vi "module api test.vi"() -> ()   [LabVIEW 2013, in "scan engine tests.lvlib"]
uses:
  scan engine tests.lvlib
  configuration/Scan Engine configuration.lvclass
  execution/Scan Engine runtime.lvclass
  <vilib>/NI/Tag Bus Module Framework/channel/channel classification.ctl
  <vilib>/NI/Tag Bus/tag/Data Type.ctl
  <vilib>/Platform/TimedLoop/XDataNode/timing_clust.ctl
  <vilib>/Platform/TimedLoop/XDataNode/nitl_modes.ctl
  <vilib>/Platform/TimedLoop/XDataNode/wakeup.ctl
  <vilib>/NI/Module Timing Source/timing source/TBM timing source.lvclass
  <vilib>/platform/TimedLoop/XDataNode/XDataNode.xnode
  <vilib>/NI/Tag Bus/tag/tag descriptor.lvclass
  <vilib>/NI/Tag Bus Module Framework/channel/TBM channel.lvclass
  <vilib>/Platform/TimedLoop/XDataNode/XDNodeRunTimeDep.lvlib
panel:
  out "Numeric":i32
  in  "stop":bool
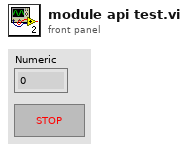
[diagram p1: front panel]
types:
  T1 = typedef "TBM channel.lvclass/channel classification.ctl" = enum16{"input data", "output data", "processing parameter", "processing result"}
  T2 = typedef "tag bus.lvlib/tag descriptor.lvclass/Data Type.ctl" = enum16{"Double", "Single", "I64", "I32", "I16", "I8", "U64", "U32", "U16", "U8", "Boolean", "String", "Array of Double", "Array of Single", "Array of I64", "Array of I32", "Array of I16", "Array of I8", "Array of U64", "Array of U32", "Array of U16", "Array of U8", "Array of Boolean", "Array of String"}
  T3 = typedef "TBM channel.lvclass/data tables.ctl" = cluster{"input data":T4, "processing parameter":T4, "processing result":T4, "output data":T4}
  T4 = typedef "tag bus.lvlib/dictionary table pair.ctl" = cluster{"data dictionary":refnum<class "data dictionary.lvclass">, "data table":T5}
  T5 = typedef "tag bus.lvlib/data table.lvlib/data table.ctl" = cluster{"Double":dbl[], "Single":sgl[], "I64":i64[], "I32":i32[], "I16":i16[], "I8":i8[], "U64":u64[], "U32":u32[], "U16":u16[], "U8":u8[], "Boolean":bool[], "String":string[], "Array of Double":cluster{"DBL Array":dbl[]}[], "Array of Single":cluster{"SGL Array":sgl[]}[], "Array of I64":cluster{"I64 Array":i64[]}[], "Array of I32":cluster{"I32 Array":i32[]}[], "Array of I16":cluster{"I16 Array":i16[]}[], "Array of I8":cluster{"I8 Array":i8[]}[], "Array of U64":cluster{"U64 Array":u64[]}[], "Array of U32":cluster{"U32 Array":u32[]}[], "Array of U16":cluster{"U16 Array":u16[]}[], "Array of U8":cluster{"U8 Array":u8[]}[], "Array of Boolean":cluster{"Boolean Array":bool[]}[], "Array of String":cluster{"String Array":string[]}[]}
  T6 = typedef "XDNodeRunTimeDep.lvlib/timing_clust.ctl" = cluster{"Expected End [f-1]":u64, "Actual End [f-1]":u64, "Finished Late? [f-1]":bool, "Expected End [i-1]":u64, "Actual End [i-1]":u64, "Finished Late? [i-1]":bool, "Expected Start [i]":u64, "Actual Start [i]":u64, "Expected Start [f]":u64, "Actual Start [f]":u64, "Source Name":string, "Structure Name":string, "Period":i64, "Deadline":i64, "Offset":i64, "Start":i64, "Priority":i32, "Timeout":i32, "Mode":T7, "Wakeup Reason":T8, "Error":errorcluster, "Source Type":string, "Secondary Source Type":string, "Global End Time":u64, "Global Start Time":u64, "Frame Duration":u64, "Iteration Duration":u64, "Assigned CPU":i32, "I/O Scan Engine Mode":u32}
  T7 = typedef "XDNodeRunTimeDep.lvlib/nitl_modes.ctl" = enum32{"No Change", "Process missed periods, maintain original phase", "Discard missed periods, maintain original phase", "Process missed periods, ignore original phase", "Discard missed periods, ignore original phase"}
  T8 = typedef "XDNodeRunTimeDep.lvlib/wakeup.ctl" = enum32{"Normal", "Aborted", "Asynchronous wakeup", "Timing source error", "Timed loop error", "Timeout"}
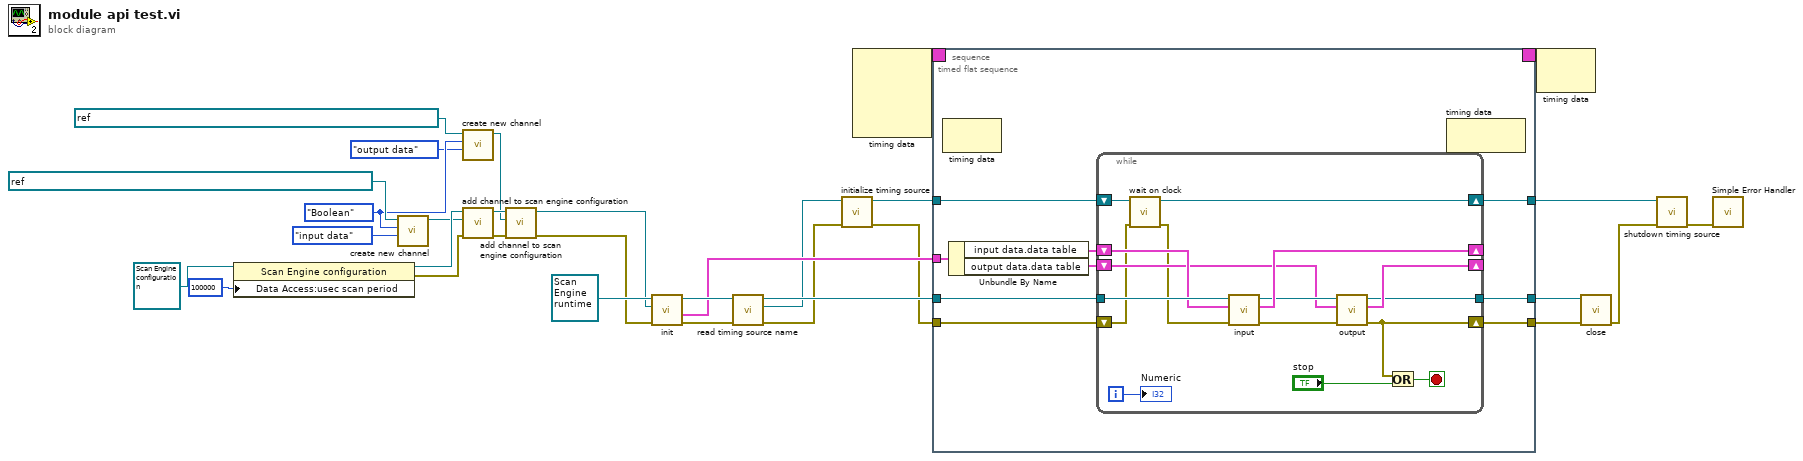
[diagram p0: block diagram]
diagram:
  w10 = Data_Type."Boolean" ("data type")
  n1 = property class="Scan Engine configuration"(reference=refnum<class "Scan Engine configuration.lvclass"> refnum ("Scan Engine configuration"), "Data Access:usec scan period"=u32 100000 ("scan period (uSec)")) -> (reference out=w7:refnum<class "Scan Engine configuration.lvclass">, error out=w6:errorcluster)  [unwired: 1 in]
  n2 = call <vilib>:"create new channel.vi"("channel classification"=channel_classification."input data", "data type"=w10, "channel name"=refnum<k21> "ni.var.io://NI-cRIO-9068-CLED/User-Defined Variables/Bool F2H" ("shared variable refnum in")) -> ("channel"=w5:refnum<class "TBM channel.lvclass">)  [unwired: 8 in]
  n3 = call <vilib>:"create new channel.vi"("channel classification"=channel_classification."output data", "data type"=w10, "channel name"=refnum<k21> "ni.var.io://NI-cRIO-9068-CLED/User-Defined Variables/Bool H2F" ("shared variable refnum in")) -> ("channel"=w3:refnum<class "TBM channel.lvclass">)  [unwired: 8 in]
  n4 = call "add channel to scan engine configuration.vi"("error in"=w6, "channel"=w5, "Scan Engine configuration in"=w7) -> ("error out"=w4:errorcluster, "Scan Engine configuration out"=w8:refnum<class "Scan Engine configuration.lvclass">)  [unwired: 7 in]
  n5 = call "add channel to scan engine configuration.vi"("error in"=w4, "channel"=w3, "Scan Engine configuration in"=w8) -> ("error out"=w1:errorcluster, "Scan Engine configuration out"=w2:refnum<class "Scan Engine configuration.lvclass">)  [unwired: 7 in]
  n6 = call-dynamic "init.vi"("error in"=w1, "TBM module configuration in"=w2, "Scan Engine runtime in"=refnum<class "Scan Engine runtime.lvclass"> refnum ("Scan Engine runtime")) -> ("error out"=w27:errorcluster, "data allocations"=w25:T3, "Scan Engine runtime out"=w28:refnum<class "Scan Engine runtime.lvclass">)  [unwired: 5 in, 1 out]
  n7 = call-dynamic "read timing source name.vi"("error in"=w27, "module in"=w28) -> ("error out"=w20:errorcluster, "timing source"=w18:refnum<class "TBM timing source.lvclass">, "module out"=w26:refnum<class "Scan Engine runtime.lvclass">)  [unwired: 7 in]
  n8 = call-dynamic "initialize timing source.vi"("error in"=w20, "timing source in"=w18) -> ("error out"=w19:errorcluster, "timing source out"=w17:refnum<class "TBM timing source.lvclass">)  [unwired: 8 in]
  n9 = node-c288() -> (w22:T6)  [unwired: 4 in]
  n10 = timed-sequence {
    timing: w22 -> [_]
    timing-out: [_] -> w21
    tunnel: w26 -> [w38]
    tunnel: w25 -> [w37]
    tunnel: [w36] -> w24
    tunnel: w19 -> [w35]
    tunnel: [w34] -> w23
    tunnel: w17 -> [w33]
    tunnel: [w32] -> w16
    n11 = timed-flat-sequence {
      tunnel: w38 -> [w47]
      tunnel: w37 -> [w46]
      tunnel: [w43] -> w36
      tunnel: w35 -> [w42]
      tunnel: [w41] -> w34
      tunnel: w33 -> [w40]
      tunnel: [w39] -> w32
      n12 = node-c288() -> ()  [unwired: 1 in, 1 out]
      n13 = Unbundle By Name(w46) -> ("input data.data table"=w45:T5, "output data.data table"=w44:T5)
      n14 = while {
        tunnel: w47 -> [w63]
        shift-right: [w61] -> _
        shift-left: w45 -> [w62]
        shift-right: [w59] -> _
        shift-left: w44 -> [w53]
        tunnel: [w57] -> w43
        shift-right: [w52] -> w41
        shift-left: w42 -> [w51]
        shift-right: [w49] -> w39
        shift-left: w40 -> [w50]
        i -> [w54]
        stop <- w55 stop-if-true
        n15 = call-dynamic "wait on clock.vi"("error in"=w51, "timing source in"=w50) -> ("error out"=w48:errorcluster, "timing source out"=w49:refnum<class "TBM timing source.lvclass">)  [unwired: 7 in, 1 out]
        n16 = call-dynamic "input.vi"("error in"=w48, "data table in"=w62, "Scan Engine runtime in"=w63) -> ("error out"=w60:errorcluster, "data table out"=w61:T5, "Scan Engine runtime out"=w58:refnum<class "Scan Engine runtime.lvclass">)  [unwired: 6 in]
        n17 = call-dynamic "output.vi"("error in"=w60, "data table in"=w53, "Scan Engine runtime in"=w58) -> ("error out"=w52:errorcluster, "data table out"=w59:T5, "Scan Engine runtime out"=w57:refnum<class "Scan Engine runtime.lvclass">)  [unwired: 6 in]
        n18 = Or(x=w52, y="stop") -> (x .or. y?=w55:bool)
        "Numeric" <- w54
      }
      n19 = node-c288() -> ()  [unwired: 1 in, 1 out]
    }
  }
  n20 = node-c288(w21) -> ()  [unwired: 1 out]
  n21 = call-dynamic "close.vi"("error in"=w23, "Scan Engine runtime in"=w24) -> ("error out"=w15:errorcluster)  [unwired: 9 in]
  n22 = call-dynamic "shutdown timing source.vi"("error in"=w15, "timing source in"=w16) -> ("error out"=w14:errorcluster)  [unwired: 8 in, 1 out]
  n23 = call <vilib>:"Simple Error Handler.vi"("error in (no error)"=w14) -> ()  [unwired: 4 in, 5 out]
